vi "Read Spectrometer Driver.lvclass.vi"(8 "error in (no error)":errorcluster, 11 "Spectrometer in":refnum<class "Spectrometer.lvclass">) -> (0 "error out":errorcluster, 2 "Spectrometer Driver.lvclass":refnum<class "Spectrometer Driver.lvclass">, 3 "Spectrometer out":refnum<class "Spectrometer.lvclass">)   [LabVIEW 2018, in "Spectrometer.lvclass"]
uses:
  Spectrometer.lvclass
  C:/github/LabActor/Instrument Actor/Instrument Actor.lvclass
  NHMFL_Core/Libraries/Instruments/Spectrometer Driver/Spectrometer Driver.lvclass
  Instrument Actor/Instrument Actor.lvclass/Instrument Actor.ctl
  Instrument Actor/Read Instrument driver.vi
  NHMFL_Core/Libraries/Instruments/Instrument Driver/Instrument Driver.lvclass
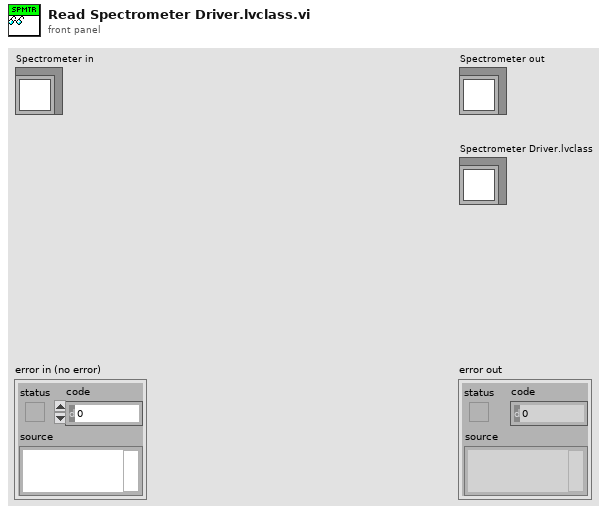
[diagram p1: front panel]
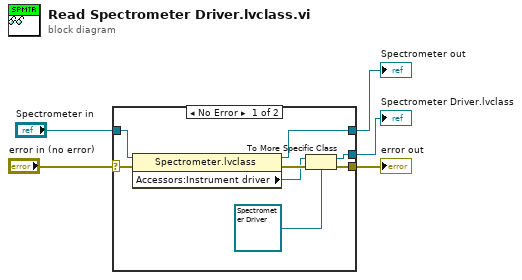
[diagram p0: block diagram]
diagram:
  n1 = case shown="No Error" "error in (no error)" {
    selector: "error in (no error)" -> [w13 w14]
    tunnel: [w9 w14] -> w4
    tunnel: [w10 w15] -> w2
    tunnel: "Spectrometer in" -> [w11 w15]
    tunnel: [w8 _] -> w1
    frame No Error {
      n2 = property class="Spectrometer.lvclass"(reference=w11, error in=w13) -> (reference out=w10:refnum<class "Spectrometer.lvclass">, error out=w12:errorcluster, "Accessors:Instrument driver"=w6:refnum<class "Instrument Driver.lvclass">)
      n3 = To More Specific Class(target class=refnum<class "Spectrometer Driver.lvclass"> refnum ("Spectrometer Driver.lvclass"), reference=w6, error in=w12) -> (specific class reference=w8:refnum<class "Spectrometer Driver.lvclass">, error out=w9:errorcluster)
    }
    frame Error {
    }
  }
  "error out" <- w4
  "Spectrometer out" <- w2
  "Spectrometer Driver.lvclass" <- w1
